vi "SetWindowParent.vi"(8 "No Error":errorcluster, 10 "Parent [SDL_Window *] (0: No Parent)":T1 format="%.0x", 11 "Window [SDL_Window *]":T1 format="%.0x") -> (0 "Error Out":errorcluster)   [LabVIEW 2026, in "SDL3.lvlib" / "Video.lvlib"]
doc: "<B>Summary</B>\nSet the window as a child of a parent window.\n\n<B>Remarks</B>\nIf the window is already the child of an existing window, it will be reparented to the new owner. Setting the parent window to NULL unparents the window and removes child window status.\n\nIf a parent window is hidden or destroyed, the operation will be recursively applied to child windows. Child windows hidden with the parent that did not have their hidden status explicitly set will be restored when the parent is shown.\n\nAttempting to set the parent of a window that is currently in the modal state will fail. Use <B>SDL_SetWindowModal()</B> to cancel the modal status before attempting to change the parent.\n\nPopup windows cannot change parents and attempts to do so will fail.\n\nSetting a parent window that is currently the sibling or descendent of the child window results in undefined behavior."
uses:
  Video.lvlib
  <vilib>/Utility/error.llb/Error Cluster From Error Code.vi
  Error/Error.lvlib
  Lib/SDL3.dll
  SDL_Window--pointer.ctl
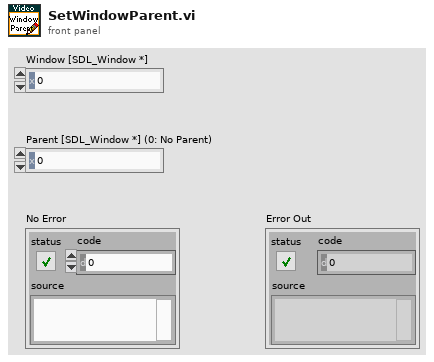
[diagram p1: front panel]
types:
  T1 = typedef "SDL3.lvlib/Video.lvlib/SDL_Window--pointer.ctl" = i64
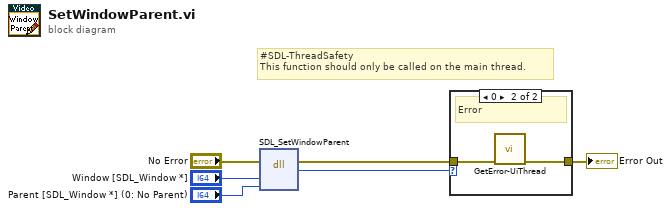
[diagram p0: block diagram]
diagram:
  # "#SDL-ThreadSafety\nThis function should only be called on the main thread."
  n1 = dll-call lib="C:/Users/saukko/Dev/LV-SDL3/Sources/SDL3/Lib/SDL3.*" fn="SDL_SetWindowParent"(error in="No Error", "window"="Window [SDL_Window *]", "parent"="Parent [SDL_Window *] (0: No Parent)") -> (error out=w3:errorcluster, "return type"=w2:i32)  [unwired: 4 in, 1 out]
  n2 = case shown="0" w2 {
    tunnel: w3 -> [w7 w9]
    tunnel: [w7 w8] -> w5
    frame Default {
      # "Ok"
    }
    frame 0 {
      # "Error"
      n3 = call "GetError-UiThread.vi"("No Error"=w9) -> ("error out"=w8:errorcluster)  [unwired: 10 in]
    }
  }
  "Error Out" <- w5
